vi "Main.vi"() -> ()   [LabVIEW 2018]
doc: "This template is for the Queued Message Handler design pattern.\n\nThe Event Handling Loop generates messages based on user interface actions.\n\nThe Message Handling Loop processes messages generated by the Event Handling Loop, or by other messages. The messages are string values, so new messages can be added easily to the Message Cases case structure in the Message Handling Loop. Each message cluster can also provide an optional value for Message Data, which is a variant that can be converted to whatever message-specific data is required."
uses:
  controls/UI Data.ctl
  support/Message Queue/Message Queue.lvlib
  support/User Event - Stop/User Event - Stop.lvlib
  support/Message Queue/Enqueue Message (Single).vi
  controls/ChangeServoPosition.ctl
  controls/EnableDisableControls.ctl
  <vilib>/Instr/_visa.llb/VISA Configure Serial Port (Instr).vi
panel:
  in  "Show Instructions":bool
  in  "Robot Arm Position":T1(radio)=enum."Position 2"
  in  "VISA resource name":refnum<visa-resource-name>="COM5"
  in  "Servo 3":i16(knob) scale=0.0..90.0
  in  "Servo 2":i16(knob) scale=0.0..90.0
  in  "INIT":bool
  in  "Servo 1":i16(knob) scale=0.0..90.0
  in  "Exit":bool
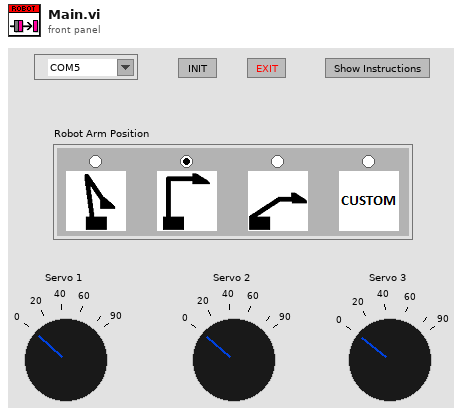
[diagram p1: front panel]
types:
  T1 = enum32{"Position 1", "Position 2", "Position 3", "Position 4"}
  T2 = typedef "UI Data.ctl" = cluster{"VISA resource name":refnum<visa-resource-name>, "\nCommunication Log Ref":refnum<file>, "Servo 1 Ctl Ref":refnum<vi>, "Servo 2 Ctl Ref":refnum<vi>, "Servo 3 Ctl Ref":refnum<vi>, "Robot Arm Position":refnum<vi>, "Position Log Ref":refnum<k34>}
  T3 = typedef "Message Queue.lvlib/All Message Queues.ctl" = cluster{"UI":refnum<queue>}
  T4 = typedef "EnableDisableControls.ctl" = cluster{"Buttons":bool, "Knobs":bool, "Servo 1 value":i16, "Servo 2 value":i16}
  T5 = enum8{"Enabled", "Disabled", "Disabled and Grayed Out"}
  T6 = typedef "ChangeServoPosition.ctl" = cluster{"Label.Text":string, "Value":i16}
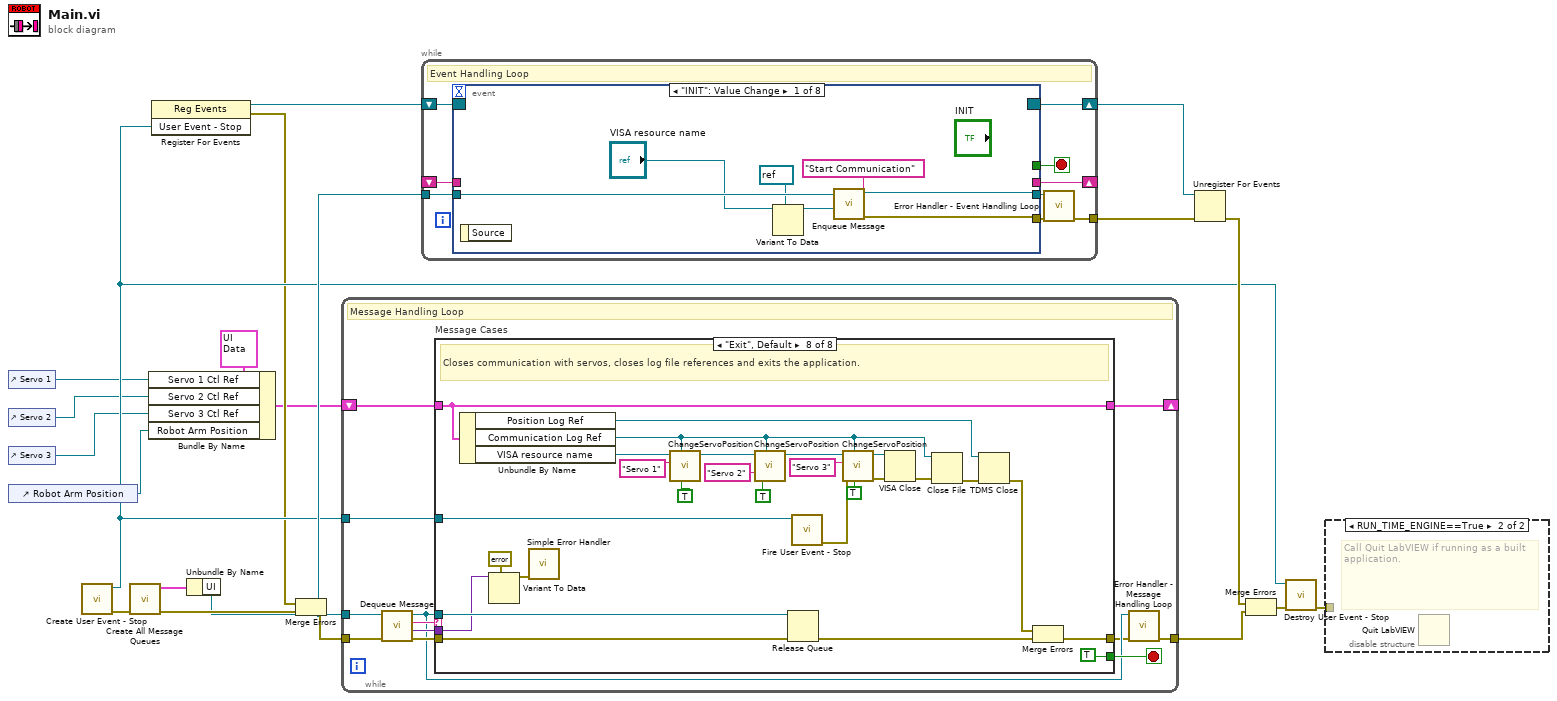
[diagram p0: block diagram]
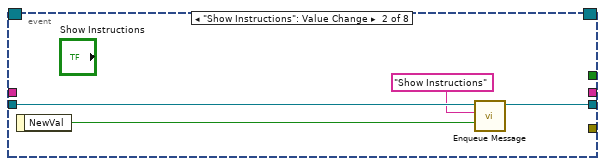
[diagram p3: hidden frame]
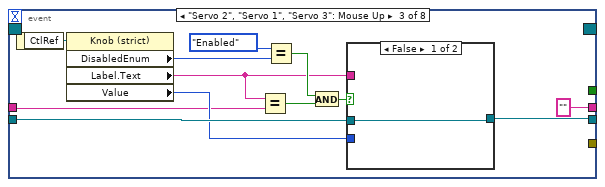
[diagram p4: hidden frame]
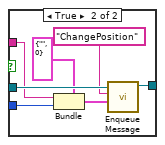
[diagram p5: hidden frame]
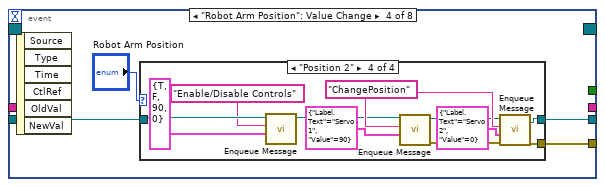
[diagram p6: hidden frame]
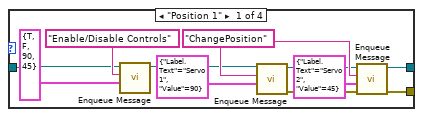
[diagram p7: hidden frame]
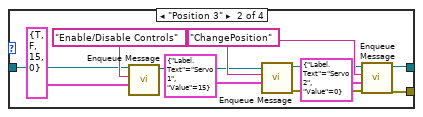
[diagram p8: hidden frame]
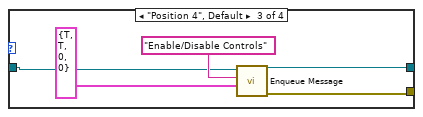
[diagram p9: hidden frame]
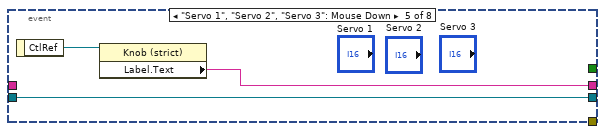
[diagram p10: hidden frame]
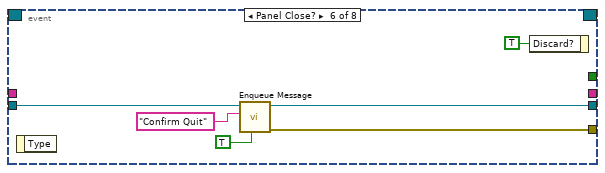
[diagram p11: hidden frame]
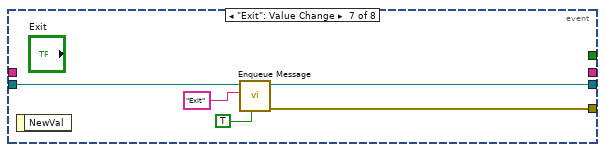
[diagram p12: hidden frame]
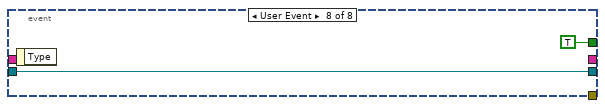
[diagram p13: hidden frame]
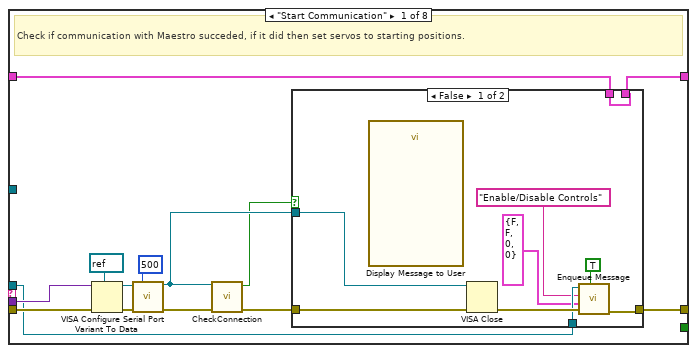
[diagram p14: hidden frame]
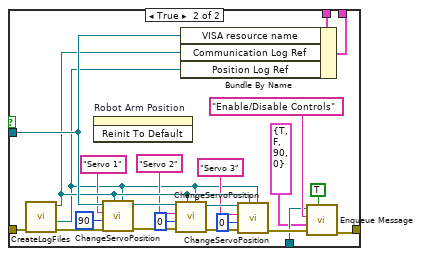
[diagram p15: hidden frame]
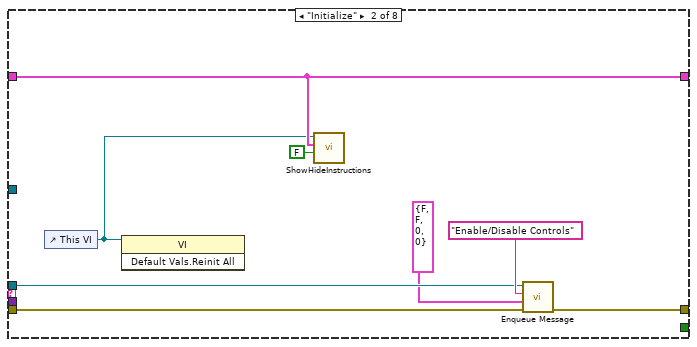
[diagram p16: hidden frame]
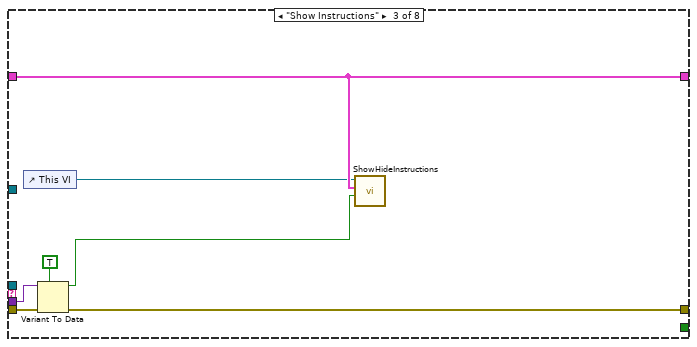
[diagram p17: hidden frame]
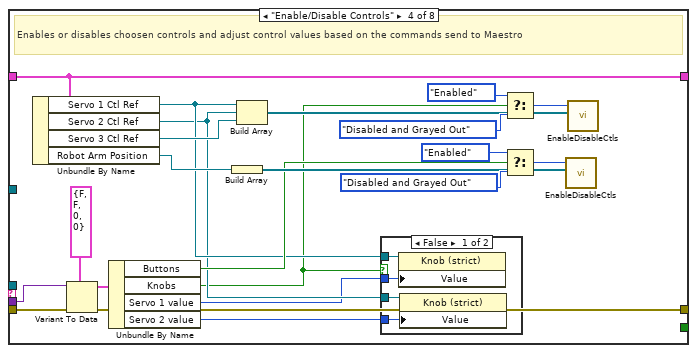
[diagram p18: hidden frame]
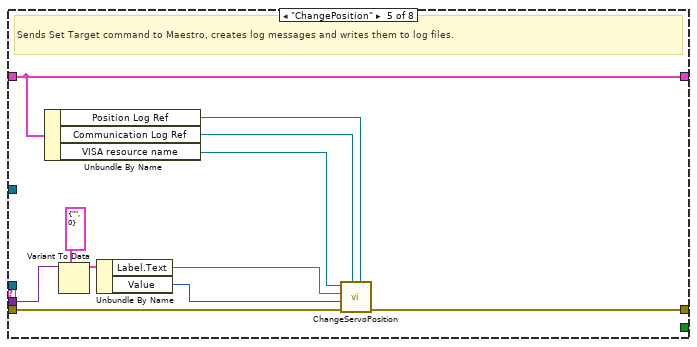
[diagram p20: hidden frame]
diagram:
  n1 = control-ref of="Servo 1"() -> (w2:refnum<vi>)
  n2 = control-ref of="Servo 2"() -> (w4:refnum<vi>)
  n3 = control-ref of="Servo 3"() -> (w3:refnum<vi>)
  n4 = control-ref of="Robot Arm Position"() -> (w1:refnum<vi>)
  n5 = call "Create User Event - Stop.vi"() -> ("error out"=w16:errorcluster, "User Event - Stop"=w9:refnum<user-event>)  [unwired: 10 in]
  n6 = call "Create All Message Queues.vi"("error in (no error)"=w16) -> ("error out"=w20:errorcluster, "Message Queues out"=w19:T3)  [unwired: 9 in]
  n7 = Bundle By Name(cluster=T2 {"VISA resource name"="", "\nCommunication Log Ref"=refnum, "Servo 1 Ctl Ref"=refnum, "Servo 2 Ctl Ref"=refnum, "Servo 3 Ctl Ref"=refnum, "Robot Arm Position"=refnum, "Position Log Ref"=refnum} ("Data Cluster"), "Servo 1 Ctl Ref"=w2, "Servo 2 Ctl Ref"=w4, "Servo 3 Ctl Ref"=w3, "Robot Arm Position"=w1) -> (w5:T2)
  n8 = register-events(w9) -> (reference out=w10:refnum<event-registration>, error out=w7:errorcluster)  [unwired: 2 in]
  n9 = Unbundle By Name(w19) -> ("UI"=w17:refnum<queue>)
  n10 = Merge Errors(w7, w20) -> (w8:errorcluster)
  n11 = while {
    tunnel: w17 -> [w24]
    shift-right: [w31] -> _
    shift-left: w5 -> [w32]
    tunnel: w9 -> [w29]
    tunnel: w8 -> [w28]
    tunnel: [w22] -> w18
    stop <- w30 stop-if-true
    # "Message Handling Loop"
    n12 = call "Dequeue Message.vi"("error in (no error)"=w28, "Message Queue"=w24) -> ("error out"=w27:errorcluster, "Message Data"=w25:variant, "Message"=w26:string, "dup Message Queue"=w23:refnum<queue>)  [unwired: 6 in]
    n13 = case "Message Cases" shown="\"Exit\", Default" w26 {
      tunnel: w23 -> [w35 w83 _ _ _ _ w140 w175]
      tunnel: w27 -> [w46 w86 w93 w111 w128 w137 w142 w149]
      tunnel: [w41 w85 w92 w110 w126 w131 w138 w172] -> w21
      tunnel: w32 -> [w38 w82 w89 w115 w130 w136 w141 w167]
      tunnel: [w36 w82 w89 w115 w130 w136 w141 w167] -> w31
      tunnel: [_ _ _ _ _ _ _ TRUE] -> w30
      tunnel: w25 -> [w45 _ w90 w112 w129 w135 _ w168]
      tunnel: w29 -> [_ _ _ _ _ _ _ w171]
      frame "Start Communication" {
        # "Check if communication with Maestro succeded, if it did then set servos to starting positions."
        n14 = Variant To Data(error in=w46, type=refnum<visa-resource-name> refnum ("VISA resource name 2"), Variant=w45) -> (data=w43:refnum<visa-resource-name>, error out=w42:errorcluster)
        n15 = call-poly "VISA Configure Serial Port"("VISA resource name"=w43, "timeout (10sec)"=u32 500, "error in (no error)"=w42) -> ("VISA resource name out"=w37:refnum<visa-resource-name>, "error out"=w34:errorcluster)  [unwired: 6 in, 5 out]
        n16 = call "CheckConnection.vi"("error in (no error)"=w34, "VISA Refnum in"=w37) -> ("error out"=w39:errorcluster, "Communication succeded?"=w33:bool)  [unwired: 8 in]
        n17 = case shown="False" w33 {
          tunnel: w39 -> [w53 w76]
          tunnel: [w51 w63] -> w41
          tunnel: w38 -> [w55 w78]
          tunnel: w37 -> [w54 w74]
          tunnel: [w55 w77] -> w36
          tunnel: w35 -> [w50 w60]
          frame False {
            n18 = call "Display Message to User"() -> ()  [unwired: 10 in, 2 out]
            n19 = VISA Close(VISA resource name=w54, error in (no error)=w53) -> (error out=w52:errorcluster)
            n20 = call-poly "Enqueue Message.vi"("Priority Message? (F)"=TRUE, "error in (no error)"=w52, "Message Data"=T4 {"Buttons"=FALSE, "Knobs"=FALSE, "Servo 1 value"=0, "Servo 2 value"=0}, "Message"="Enable/Disable Controls", "Message Queue"=w50) -> ("error out"=w51:errorcluster)  [unwired: 5 in, 1 out]
          }
          frame True {
            n21 = call "CreateLogFiles.vi"("error in (no error)"=w76) -> ("error out"=w75:errorcluster, "Tdms log file"=w57:refnum<k34>, "Txt log file"=w71:refnum<file>)  [unwired: 8 in]
            n22 = invoke on="Robot Arm Position" class="RadioBtnsControl (strict)" method="Reinit To Default"() -> ()  [unwired: 3 in, 3 out]
            n23 = call "ChangeServoPosition.vi"("Position Log Ref"=w57, "Communication Log Ref"=w71, "error in (no error)"=w75, "Value"=i16 90, "Label.Text"="Servo 1", "VISA Refnum in"=w74) -> ("error out"=w73:errorcluster, "VISA resource name out"=w69:refnum<visa-resource-name>)  [unwired: 4 in]
            n24 = call "ChangeServoPosition.vi"("Position Log Ref"=w57, "Communication Log Ref"=w71, "error in (no error)"=w73, "Value"=i16 0, "Label.Text"="Servo 2", "VISA Refnum in"=w69) -> ("error out"=w72:errorcluster, "VISA resource name out"=w70:refnum<visa-resource-name>)  [unwired: 4 in]
            n25 = Bundle By Name(cluster=w78, "VISA resource name"=w74, "Communication Log Ref"=w71, "Position Log Ref"=w57) -> (w77:T2)
            n26 = call "ChangeServoPosition.vi"("Position Log Ref"=w57, "Communication Log Ref"=w71, "error in (no error)"=w72, "Value"=i16 0, "Label.Text"="Servo 3", "VISA Refnum in"=w70) -> ("error out"=w64:errorcluster)  [unwired: 4 in, 1 out]
            n27 = call-poly "Enqueue Message.vi"("Priority Message? (F)"=TRUE, "error in (no error)"=w64, "Message Data"=T4 {"Buttons"=TRUE, "Knobs"=FALSE, "Servo 1 value"=90, "Servo 2 value"=0}, "Message"="Enable/Disable Controls", "Message Queue"=w60) -> ("error out"=w63:errorcluster)  [unwired: 5 in, 1 out]
          }
        }
      }
      frame "Initialize" {
        n28 = control-ref of="This VI"() -> (w81:refnum<vi>)
        n29 = invoke class="VI" method="Default Vals.Reinit All"(reference=w81) -> ()  [unwired: 2 in, 3 out]
        n30 = call "ShowHideInstructions.vi"("Show/Hide"=FALSE ("Boolean"), "Data Cluster"=w82, "VI in"=w81) -> ()  [unwired: 9 in]
        n31 = call-poly "Enqueue Message.vi"("error in (no error)"=w86, "Message Data"=T4 {"Buttons"=FALSE, "Knobs"=FALSE, "Servo 1 value"=0, "Servo 2 value"=0}, "Message"="Enable/Disable Controls", "Message Queue"=w83) -> ("error out"=w85:errorcluster)  [unwired: 6 in, 1 out]
      }
      frame "Show Instructions" {
        n32 = control-ref of="This VI"() -> (w87:refnum<vi>)
        n33 = Variant To Data(error in=w93, type=TRUE, Variant=w90) -> (data=w88:bool, error out=w92:errorcluster)
        n34 = call "ShowHideInstructions.vi"("Show/Hide"=w88, "Data Cluster"=w89, "VI in"=w87) -> ()  [unwired: 9 in]
      }
      frame "Enable/Disable Controls" {
        # "Enables or disables choosen controls and adjust control values based on the commands send to Maestro"
        n35 = Unbundle By Name(w115) -> ("Servo 1 Ctl Ref"=w99:refnum<vi>, "Servo 2 Ctl Ref"=w98:refnum<vi>, "Servo 3 Ctl Ref"=w114:refnum<vi>, "Robot Arm Position"=w113:refnum<vi>)
        n36 = Variant To Data(error in=w111, type=T4 {"Buttons"=FALSE, "Knobs"=FALSE, "Servo 1 value"=0, "Servo 2 value"=0}, Variant=w112) -> (data=w109:T4, error out=w110:errorcluster)
        n37 = Unbundle By Name(w109) -> ("Buttons"=w100:bool, "Knobs"=w95:bool, "Servo 1 value"=w97:i16, "Servo 2 value"=w96:i16)
        n38 = Build Array(w113) -> (w101:refnum<vi>[])
        n39 = Build Array(w99, w98, w114) -> (w102:refnum<vi>[])
        n40 = case shown="False" w95 {
          tunnel: w99 -> [w119 _]
          tunnel: w98 -> [w118 _]
          tunnel: w97 -> [w117 _]
          tunnel: w96 -> [w116 _]
          frame False {
            n41 = property class="Knob (strict)"(reference=w119, "Value"=w117) -> ()  [unwired: 1 in, 2 out]
            n42 = property class="Knob (strict)"(reference=w118, "Value"=w116) -> ()  [unwired: 1 in, 2 out]
          }
          frame True {
          }
        }
        n43 = Select(t=T5."Enabled" ("Enable/Disable"), s=w95, f=T5."Disabled and Grayed Out" ("Enable/Disable")) -> (s? t:f=w104:T5)
        n44 = Select(t=T5."Enabled" ("Enable/Disable"), s=w100, f=T5."Disabled and Grayed Out" ("Enable/Disable")) -> (s? t:f=w103:T5)
        n45 = call "EnableDisableCtls.vi"("Ctls array"=w101, "Enable/Disable"=w103) -> ()  [unwired: 10 in]
        n46 = call "EnableDisableCtls.vi"("Ctls array"=w102, "Enable/Disable"=w104) -> ()  [unwired: 10 in]
      }
      frame "ChangePosition" {
        # "Sends Set Target command to Maestro, creates log messages and writes them to log files."
        n47 = Unbundle By Name(w130) -> ("Position Log Ref"=w121:refnum<k34>, "Communication Log Ref"=w122:refnum<file>, "VISA resource name"=w123:refnum<visa-resource-name>)
        n48 = Variant To Data(type=T6 {"Label.Text"="", "Value"=0}, Variant=w129) -> (data=w127:T6)  [unwired: 1 in, 1 out]
        n49 = Unbundle By Name(w127) -> ("Label.Text"=w124:string, "Value"=w125:i16)
        n50 = call "ChangeServoPosition.vi"("Position Log Ref"=w121, "Communication Log Ref"=w122, "error in (no error)"=w128, "Value"=w125, "Label.Text"=w124, "VISA Refnum in"=w123) -> ("error out"=w126:errorcluster)  [unwired: 4 in, 1 out]
      }
      frame "Error" {
        # "Error - Display an error dialog. This message is sent by the \"Error Handler\" VIs at the end of other loops in this application."
        n51 = Variant To Data(error in=w137, type=errorcluster {"status"=FALSE, "code"=0, "source"=""} ("error constant"), Variant=w135) -> (data=w133:errorcluster, error out=w132:errorcluster)
        n52 = call <vilib>:"Simple Error Handler.vi"("error in (no error)"=w133) -> ()  [unwired: 4 in, 5 out]
        n53 = Merge Errors(w132) -> (w131:errorcluster)
      }
      frame "Confirm Quit" {
        # "Confirm Quit - Message that can confirm whether or not the user wants to exit the application."
        n54 = call "Display Message to User2"() -> ("Yes"=w139:bool)  [unwired: 10 in, 1 out]
        n55 = case shown="True" w139 {
          tunnel: w142 -> [w143 w148]
          tunnel: [w143 w147] -> w138
          tunnel: w140 -> [_ w146]
          frame False {
          }
          frame True {
            n56 = call-poly "Enqueue Message.vi"("Priority Message? (F)"=TRUE, "error in (no error)"=w148, "Message"="Exit", "Message Queue"=w146) -> ("error out"=w147:errorcluster)  [unwired: 6 in, 1 out]
          }
        }
      }
      frame "Exit", Default {
        # "Closes communication with servos, closes log file references and exits the application."
        n57 = Unbundle By Name(w167) -> ("Position Log Ref"=w150:refnum<k34>, "Communication Log Ref"=w159:refnum<file>, "VISA resource name"=w162:refnum<visa-resource-name>)
        n58 = Variant To Data(type=errorcluster {"status"=FALSE, "code"=0, "source"=""} ("error constant"), Variant=w168) -> (data=w169:errorcluster)  [unwired: 1 in, 1 out]
        n59 = call <vilib>:"Simple Error Handler.vi"("error in (no error)"=w169) -> ()  [unwired: 4 in, 5 out]
        n60 = call "ChangeServoPosition.vi"("Close communication"=TRUE, "Communication Log Ref"=w159, "Label.Text"="Servo 1", "VISA Refnum in"=w162) -> ("VISA resource name out"=w161:refnum<visa-resource-name>)  [unwired: 6 in, 1 out]
        n61 = call "ChangeServoPosition.vi"("Close communication"=TRUE, "Communication Log Ref"=w159, "Label.Text"="Servo 2", "VISA Refnum in"=w161) -> ("VISA resource name out"=w160:refnum<visa-resource-name>)  [unwired: 6 in, 1 out]
        n62 = Release Queue(queue=w175, error in (no error)=w149) -> (error out=w173:errorcluster)  [unwired: 1 in, 2 out]
        n63 = call "Fire User Event - Stop.vi"("User Event - Stop"=w171) -> ("error out"=w153:errorcluster)  [unwired: 10 in]
        n64 = call "ChangeServoPosition.vi"("Close communication"=TRUE, "Communication Log Ref"=w159, "error in (no error)"=w153, "Label.Text"="Servo 3", "VISA Refnum in"=w160) -> ("error out"=w164:errorcluster, "VISA resource name out"=w163:refnum<visa-resource-name>)  [unwired: 5 in]
        n65 = VISA Close(VISA resource name=w163, error in (no error)=w164) -> (error out=w154:errorcluster)
        n66 = Close File(refnum=w159, error in=w154) -> (error out=w152:errorcluster)  [unwired: 1 out]
        n67 = TDMS Close(8:w152, 11:w150) -> (0:w151:errorcluster)  [unwired: 1 out]
        n68 = Merge Errors(w151, w173) -> (w172:errorcluster)
      }
    }
    n69 = call "Error Handler - Message Handling Loop.vi"("error in (no error)"=w21, "Message Queue"=w23) -> ("dup error in"=w22:errorcluster)  [unwired: 8 in, 1 out]
  }
  n70 = while {
    tunnel: w17 -> [w184]
    shift-right: [w182] -> w13
    shift-left: w10 -> [w183]
    tunnel: [w178] -> w11
    shift-right: [w177] -> _
    shift-left: _ -> [w176]
    stop <- w180 stop-if-true
    # "Event Handling Loop"
    n71 = event shown="[0] \"INIT\": Value Change" {
      selector: w183 -> [_ _ _ _ _ _ _ _]
      dyn-events: [_ _ _ _ _ _ _ _] -> w182
      timeout: _ -> [_ _ _ _ _ _ _ _]
      tunnel: [_ _ _ _ _ _ _ TRUE ("Discard?")] -> w180
      tunnel: w184 -> [w190 w195 w207 w218 w260 w265 w271 w273]
      tunnel: [w185 _ _ w216 _ w264 w270 _] -> w181
      tunnel: [w189 w194 w206 w217 w260 w263 w269 w273] -> w179
      tunnel: [_ _ "" ("Label.Text") _ w258 _ _ _] -> w177
      tunnel: w176 -> [_ _ w197 _ _ _ _ _]
      event "INIT": Value Change {
        n72 = event-data() -> ()  [unwired: 1 in, 1 out]
        n73 = Variant To Data(type=refnum<visa-resource-name> refnum ("VISA resource name 2"), Variant="VISA resource name") -> (data=w188:refnum<visa-resource-name>)  [unwired: 1 in, 1 out]
        n74 = call-poly "Enqueue Message.vi"("Message Data"=w188, "Message"="Start Communication", "Message Queue"=w190) -> ("error out"=w185:errorcluster, "dup Message Queue"=w189:refnum<queue>)  [unwired: 7 in]
      }
      event "Show Instructions": Value Change {
        n75 = event-data() -> ("NewVal"=w192:bool)  [unwired: 1 in]
        n76 = call-poly "Enqueue Message.vi"("Message Data"=w192, "Message"="Show Instructions", "Message Queue"=w195) -> ("dup Message Queue"=w194:refnum<queue>)  [unwired: 7 in, 1 out]
      }
      event "Servo 2", "Servo 1", "Servo 3": Mouse Up {
        n77 = event-data() -> ("CtlRef"=w204:refnum<vi>)  [unwired: 1 in]
        n78 = property class="Knob (strict)"(reference=w204) -> ("DisabledEnum"=w202:T5, "Label.Text"=w196:string, "Value"=w203:i16)  [unwired: 1 in, 2 out]
        n79 = Equal?(x=w196, y=w197) -> (x = y?=w200:bool)
        n80 = Equal?(x=T5."Enabled" ("Disabled"), y=w202) -> (x = y?=w199:bool)
        n81 = And(x=w199, y=w200) -> (x .and. y?=w198:bool)
        n82 = case shown="False" w198 {
          tunnel: w207 -> [w208 w215]
          tunnel: [w208 w214] -> w206
          tunnel: w203 -> [_ w212]
          tunnel: w196 -> [_ w211]
          frame False {
          }
          frame True {
            n83 = Bundle(cluster=T6 {"Label.Text"="", "Value"=0}, "Label.Text"=w211, "Value"=w212) -> (w210:T6)
            n84 = call-poly "Enqueue Message.vi"("Message Data"=w210, "Message"="ChangePosition", "Message Queue"=w215) -> ("dup Message Queue"=w214:refnum<queue>)  [unwired: 7 in, 1 out]
          }
        }
      }
      event "Robot Arm Position": Value Change {
        n85 = event-data() -> ()  [unwired: 1 in, 6 out]
        n86 = case shown="\"Position 2\"" "Robot Arm Position" {
          tunnel: w218 -> [w224 w235 w245 w252]
          tunnel: [w228 w238 w243 w254] -> w217
          tunnel: [w227 w237 w244 w253] -> w216
          frame "Position 1" {
            w230 = "ChangePosition" ("Message")
            n87 = call-poly "Enqueue Message.vi"("Message Data"=T4 {"Buttons"=TRUE, "Knobs"=FALSE, "Servo 1 value"=90, "Servo 2 value"=45}, "Message"="Enable/Disable Controls", "Message Queue"=w224) -> ("dup Message Queue"=w223:refnum<queue>)  [unwired: 7 in, 1 out]
            n88 = call-poly "Enqueue Message.vi"("Message Data"=T6 {"Label.Text"="Servo 1", "Value"=90}, "Message"=w230, "Message Queue"=w223) -> ("error out"=w226:errorcluster, "dup Message Queue"=w229:refnum<queue>)  [unwired: 7 in]
            n89 = call-poly "Enqueue Message.vi"("error in (no error)"=w226, "Message Data"=T6 {"Label.Text"="Servo 2", "Value"=45}, "Message"=w230, "Message Queue"=w229) -> ("error out"=w227:errorcluster, "dup Message Queue"=w228:refnum<queue>)  [unwired: 6 in]
          }
          frame "Position 3" {
            w241 = "ChangePosition" ("Message")
            n90 = call-poly "Enqueue Message.vi"("Message Data"=T4 {"Buttons"=TRUE, "Knobs"=FALSE, "Servo 1 value"=15, "Servo 2 value"=0}, "Message"="Enable/Disable Controls", "Message Queue"=w235) -> ("dup Message Queue"=w234:refnum<queue>)  [unwired: 7 in, 1 out]
            n91 = call-poly "Enqueue Message.vi"("Message Data"=T6 {"Label.Text"="Servo 1", "Value"=15}, "Message"=w241, "Message Queue"=w234) -> ("error out"=w239:errorcluster, "dup Message Queue"=w240:refnum<queue>)  [unwired: 7 in]
            n92 = call-poly "Enqueue Message.vi"("error in (no error)"=w239, "Message Data"=T6 {"Label.Text"="Servo 2", "Value"=0}, "Message"=w241, "Message Queue"=w240) -> ("error out"=w237:errorcluster, "dup Message Queue"=w238:refnum<queue>)  [unwired: 6 in]
          }
          frame "Position 4", Default {
            n93 = call-poly "Enqueue Message.vi"("Message Data"=T4 {"Buttons"=TRUE, "Knobs"=TRUE, "Servo 1 value"=0, "Servo 2 value"=0}, "Message"="Enable/Disable Controls", "Message Queue"=w245) -> ("error out"=w244:errorcluster, "dup Message Queue"=w243:refnum<queue>)  [unwired: 7 in]
          }
          frame "Position 2" {
            w257 = "ChangePosition" ("Message")
            n94 = call-poly "Enqueue Message.vi"("Message Data"=T4 {"Buttons"=TRUE, "Knobs"=FALSE, "Servo 1 value"=90, "Servo 2 value"=0}, "Message"="Enable/Disable Controls", "Message Queue"=w252) -> ("dup Message Queue"=w251:refnum<queue>)  [unwired: 7 in, 1 out]
            n95 = call-poly "Enqueue Message.vi"("Message Data"=T6 {"Label.Text"="Servo 1", "Value"=90}, "Message"=w257, "Message Queue"=w251) -> ("error out"=w255:errorcluster, "dup Message Queue"=w256:refnum<queue>)  [unwired: 7 in]
            n96 = call-poly "Enqueue Message.vi"("error in (no error)"=w255, "Message Data"=T6 {"Label.Text"="Servo 2", "Value"=0}, "Message"=w257, "Message Queue"=w256) -> ("error out"=w253:errorcluster, "dup Message Queue"=w254:refnum<queue>)  [unwired: 6 in]
          }
        }
      }
      event "Servo 1", "Servo 2", "Servo 3": Mouse Down {
        n97 = event-data() -> ("CtlRef"=w259:refnum<vi>)  [unwired: 1 in]
        n98 = property class="Knob (strict)"(reference=w259) -> ("Label.Text"=w258:string)  [unwired: 1 in, 2 out]
      }
      event Panel Close? {
        n99 = event-data() -> ()  [unwired: 1 in, 1 out]
        n100 = call-poly "Enqueue Message.vi"("Priority Message? (F)"=TRUE, "Message"="Confirm Quit", "Message Queue"=w265) -> ("error out"=w264:errorcluster, "dup Message Queue"=w263:refnum<queue>)  [unwired: 7 in]
        n101 = event-data("Discard?"=TRUE) -> ()  [unwired: 1 in, 1 out]
      }
      event "Exit": Value Change {
        n102 = event-data() -> ()  [unwired: 1 in, 1 out]
        n103 = call-poly "Enqueue Message.vi"("Priority Message? (F)"=TRUE, "Message"="Exit", "Message Queue"=w271) -> ("error out"=w270:errorcluster, "dup Message Queue"=w269:refnum<queue>)  [unwired: 7 in]
      }
      event User Event {
        n104 = event-data() -> ()  [unwired: 1 in, 1 out]
      }
    }
    n105 = call "Error Handler - Event Handling Loop.vi"("error in (no error)"=w181, "Message Queue"=w179) -> ("dup error in"=w178:errorcluster)  [unwired: 8 in, 1 out]
  }
  n106 = Unregister For Events(event registration refnum=w13, error in=w11) -> (error out=w14:errorcluster)
  n107 = Merge Errors(w14, w18) -> (w15:errorcluster)
  n108 = call "Destroy User Event - Stop.vi"("error in (no error)"=w15, "User Event - Stop"=w9) -> ("error out"=w12:errorcluster)  [unwired: 9 in]
  n109 = disable-structure shown="RUN_TIME_ENGINE==True" {
    disable-tunnel: w12 -> [_ _]
    frame condition #0 (active) {
    }
    frame condition #1 {
      # "Call Quit LabVIEW if running as a built application."
      n110 = Quit LabVIEW() -> ()  [unwired: 1 in]
    }
  }
